vi "niRFUtil RFHS Channelizer ChannelizerErrorToText.vi"(0 "Error List":T1, 5 "Additional Info":i32, 7 "Additional info":string, 11 "error in (no error)":errorcluster) -> (15 "error out":errorcluster)   [LabVIEW 2015, in "niRFUtil.lvlib"]
uses:
  niRFUtil.lvlib
  Includes/niRFUtil RFHS Channelizer ChannelizerErrors.ctl
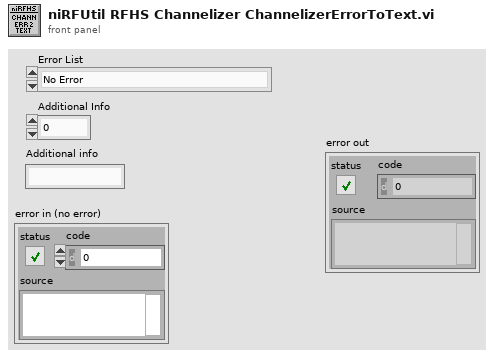
[diagram p1: front panel]
types:
  T1 = typedef "niRFUtil.lvlib/niRFUtil RFHS Channelizer ChannelizerErrors.ctl" = enum32{"No Error", "Invalid Channel", "Internal Error", "Invalid Channel fs", "Invalid Phase Shift", "Invalid fs", "Invalid Number Of Channles", "Invalid FFT Channel fs", "Invalid Resampler Channel fs", "Not a 15kHz Multiple", "Invalid Channel fc", "Invalid passBW/stopBW", "Coerced Rejection", "Requires Internal Buffer", "Duplicated Destination Channel Name", "Configuration Format Error", "Illegal Execution state", "DLL not found", "DLL loading failure", "AVX instruction failure"}
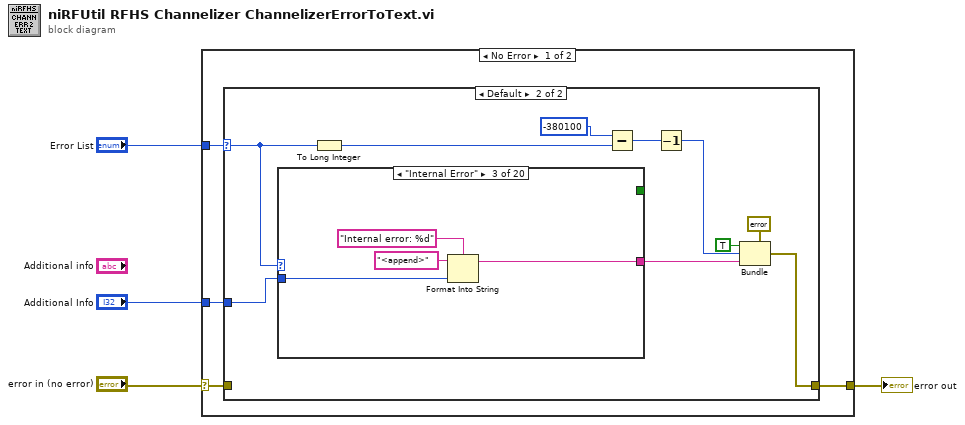
[diagram p0: block diagram]
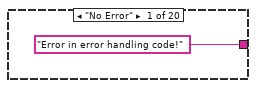
[diagram p3: hidden frame]
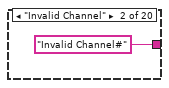
[diagram p4: hidden frame]
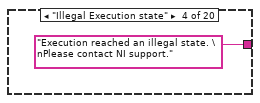
[diagram p5: hidden frame]
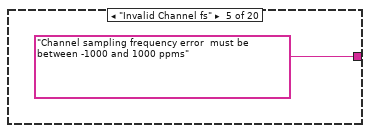
[diagram p6: hidden frame]
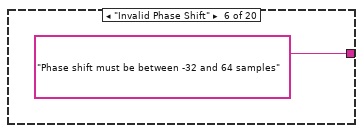
[diagram p7: hidden frame]
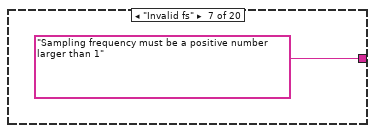
[diagram p8: hidden frame]
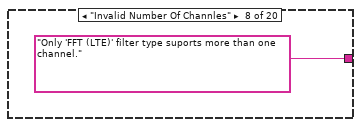
[diagram p9: hidden frame]
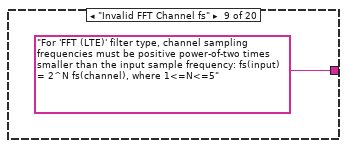
[diagram p10: hidden frame]
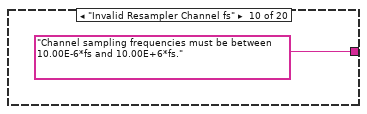
[diagram p11: hidden frame]
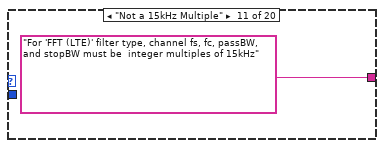
[diagram p12: hidden frame]
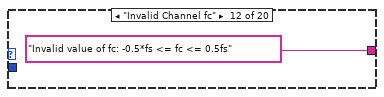
[diagram p13: hidden frame]
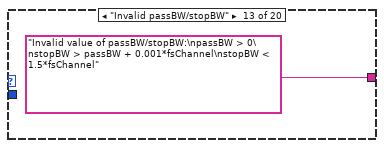
[diagram p14: hidden frame]
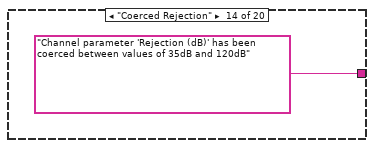
[diagram p15: hidden frame]
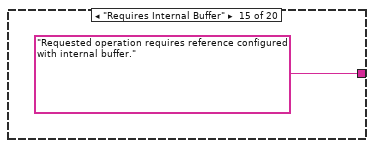
[diagram p16: hidden frame]
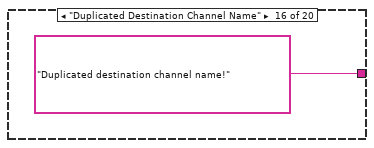
[diagram p17: hidden frame]
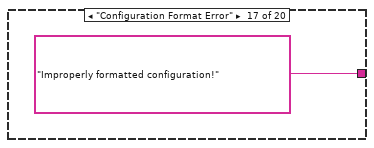
[diagram p18: hidden frame]
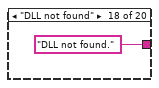
[diagram p19: hidden frame]
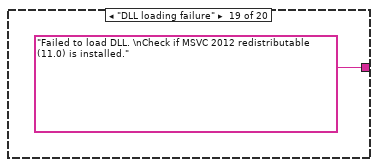
[diagram p20: hidden frame]
diagram:
  n1 = case shown="No Error" "error in (no error)" {
    selector: "error in (no error)" -> [w6 w44]
    tunnel: "Additional Info" -> [w8 _]
    tunnel: "Error List" -> [w7 _]
    tunnel: [w5 w44] -> w1
    frame No Error {
      n2 = case shown="Default" w7 {
        selector: w7 -> [_ w15]
        tunnel: w8 -> [_ w17]
        tunnel: w6 -> [w9 _]
        tunnel: [w9 w10] -> w5
        frame "No Error" {
        }
        frame Default {
          n3 = case shown="\"Internal Error\"" w15 {
            tunnel: ["Error in error handling code!" "Invalid Channel#" w23 "Execution reached an illegal state. \nPlease contact NI support." ("source") "Channel sampling frequency error  must be between -1000 and 1000 ppms" ("source") "Phase shift must be between -32 and 64 samples" ("source") "Sampling frequency must be a positive number larger than 1" ("source") "Only 'FFT (LTE)' filter type suports more than one channel." ("source") "For 'FFT (LTE)' filter type, channel sampling frequencies must be positive power-of-two times  smaller than the input sample frequency: fs(input) = 2^N fs(channel), where 1<=N<=5" ("source") "Channel sampling frequencies must be between 10.00E-6*fs and 10.00E+6*fs." ("source") "For 'FFT (LTE)' filter type, channel fs, fc, passBW, and stopBW must be  integer multiples of 15kHz" ("source") "Invalid value of fc: -0.5*fs <= fc <= 0.5fs" ("source") "Invalid value of passBW/stopBW:\npassBW > 0\nstopBW > passBW + 0.001*fsChannel\nstopBW < 1.5*fsChannel" ("source") "Channel parameter 'Rejection (dB)' has been coerced between values of 35dB and 120dB" ("source") "Requested operation requires reference configured with internal buffer." ("source") "Duplicated destination channel name!" ("source") "Improperly formatted configuration!" ("source") "DLL not found." ("source") "Failed to load DLL. \nCheck if MSVC 2012 redistributable (11.0) is installed." ("source") "Bogus AVX unit.\nThe framework will fall back to slower non-AVX implementation." ("source")] -> w11
            tunnel: w17 -> [_ _ w24 _ _ _ _ _ _ _ _ _ _ _ _ _ _ _ _ _]
            tunnel: [_ _ _ _ _ _ _ _ _ _ _ _ _ _ _ _ _ _ _ TRUE ("is warning? (False)")] -> _
            frame "No Error" {
            }
            frame "Invalid Channel" {
            }
            frame "Internal Error" {
              n4 = Format Into String(format string="Internal error: %d", initial string="<append>", w24) -> (resulting string=w23:string)  [unwired: 1 in, 1 out]
            }
            frame "Illegal Execution state" {
            }
            frame "Invalid Channel fs" {
            }
            frame "Invalid Phase Shift" {
            }
            frame "Invalid fs" {
            }
            frame "Invalid Number Of Channles" {
            }
            frame "Invalid FFT Channel fs" {
            }
            frame "Invalid Resampler Channel fs" {
            }
            frame "Not a 15kHz Multiple" {
            }
            frame "Invalid Channel fc" {
            }
            frame "Invalid passBW/stopBW" {
            }
            frame "Coerced Rejection" {
            }
            frame "Requires Internal Buffer" {
            }
            frame "Duplicated Destination Channel Name" {
            }
            frame "Configuration Format Error" {
            }
            frame "DLL not found" {
            }
            frame "DLL loading failure" {
            }
            frame "AVX instruction failure" {
            }
          }
          n5 = To Long Integer(number=w15) -> (32bit integer=w16:i32)
          n6 = Subtract(x=-380100 ("code"), y=w16) -> (x-y=w18:i32)
          n7 = Decrement(x=w18) -> (x-1=w12:i32)
          n8 = Bundle(cluster=errorcluster {"status"=FALSE, "code"=0, "source"=""} ("error constant"), "status"=TRUE, "code"=w12, "source"=w11) -> (w10:errorcluster)
        }
      }
    }
    frame Error {
    }
  }
  "error out" <- w1
